vi "getfIRF.vi"(8 "error in (no error)":errorcluster, 11 "LaguerreDeconEngineClass in":refnum<class "LaguerreDeconEngineClass.lvclass">) -> (0 "error out":errorcluster, 2 "fIRF":dbl[](array[numeric]), 3 "LaguerreDeconEngineClass out":refnum<class "LaguerreDeconEngineClass.lvclass">)   [LabVIEW 2024, in "LaguerreDeconEngineClass.lvclass"]
uses:
  LaguerreDeconEngineClass.lvclass
  LaguerreDeconEngineClass.lvclass/LaguerreDeconEngineClass.ctl
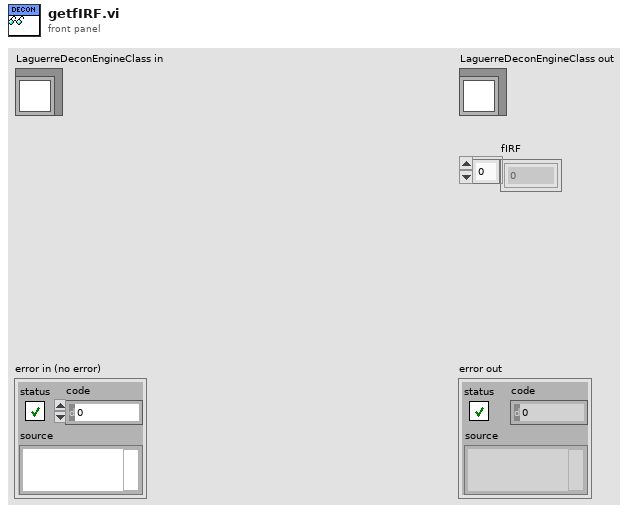
[diagram p1: front panel]
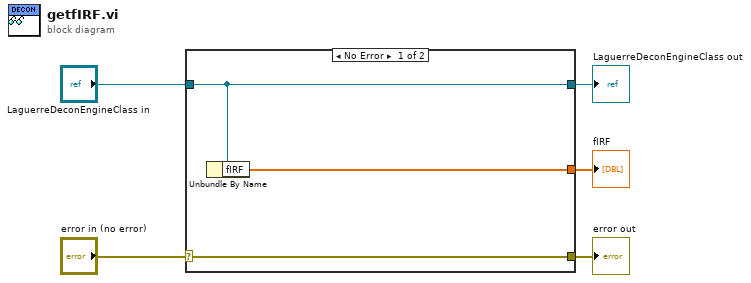
[diagram p0: block diagram]
diagram:
  n1 = case shown="No Error" "error in (no error)" {
    selector: "error in (no error)" -> [w8 w9]
    tunnel: [w8 w9] -> w4
    tunnel: [w7 w10] -> w2
    tunnel: "LaguerreDeconEngineClass in" -> [w7 w10]
    tunnel: [w6 _] -> w1
    frame No Error {
      n2 = Unbundle By Name(w7) -> ("fIRF"=w6:dbl[])
    }
    frame Error {
    }
  }
  "error out" <- w4
  "LaguerreDeconEngineClass out" <- w2
  "fIRF" <- w1
